vi "Post-Build Action.vi"(5 "Files Generated by Build":path[](array[path]), 6 "Top Level/Always Included VIs":path[](array[path]), 7 "Destination Path":path, 8 "error in (no error)":errorcluster, 9 "Target Name":string, 10 "Build Specification Name":string, 11 "Project Path":path) -> (0 "error out":errorcluster)   [LabVIEW 2017]
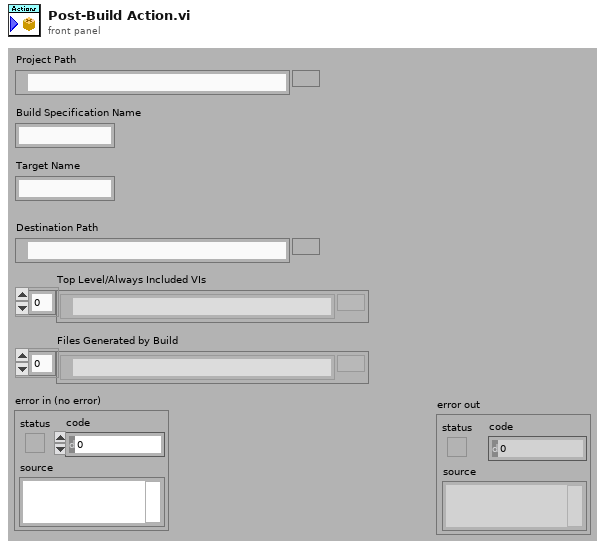
[diagram p1: front panel]
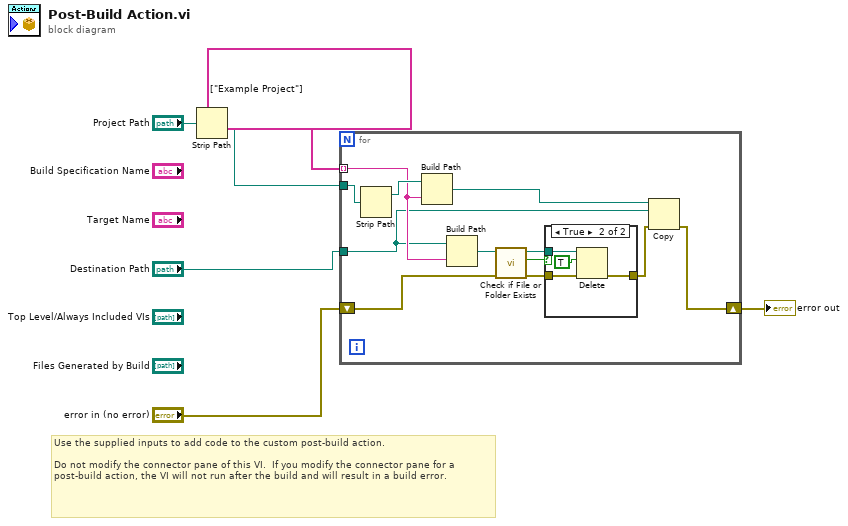
[diagram p0: block diagram]
diagram:
  # "Use the supplied inputs to add code to the custom post-build action.\n\nDo not modify the connector pane of this VI.  If you modify the connector pane for a post-build action, the VI will not run after the build and will result in a build error."
  n1 = Strip Path(path="Project Path") -> (stripped path=w4:path)  [unwired: 1 out]
  n2 = for {
    tunnel: string[] ["Example Project"] -> [w9] mode=indexing
    tunnel: w4 -> [w18]
    tunnel: "Destination Path" -> [w7]
    shift-right: [w15] -> w1
    shift-left: "error in (no error)" -> [w12]
    n3 = Strip Path(path=w18) -> (stripped path=w17:path)  [unwired: 1 out]
    n4 = Build Path(base path=w17, name or relative path=w9) -> (appended path=w16:path)
    n5 = Build Path(base path=w7, name or relative path=w9) -> (appended path=w8:path)
    n6 = call <vilib>:"Check if File or Folder Exists.vi"("error in (no error)"=w12, "path"=w8) -> ("error out"=w11:errorcluster, "file or folder exists?"=w13:bool, "dup path"=w14:path)  [unwired: 7 in]
    n7 = case shown="True" w13 {
      tunnel: w14 -> [_ w23]
      tunnel: w11 -> [w19 w22]
      tunnel: [w19 w21] -> w10
      frame False {
      }
      frame True {
        n8 = Delete(path (use dialog)=w23, entire hierarchy (F)=TRUE, error in=w22) -> (error out=w21:errorcluster)  [unwired: 2 in, 2 out]
      }
    }
    n9 = Copy(8:w10, 10:w7, 11:w16) -> (0:w15:errorcluster)  [unwired: 2 in, 2 out]
  }
  "error out" <- w1
